vi "Main.vi"() -> ()   [LabVIEW 2012]
uses:
  <userlib>/DAQNavi Polymorphic VI/create/DAQNavi Create Channel(AI-Voltage).vi
  <userlib>/DAQNavi Polymorphic VI/configure/timing/DAQNavi Timing(AI Convert Clock).vi
  <userlib>/DAQNavi Polymorphic VI/read/DAQNavi Read (Analog 1D U16 NChan NSamp).vi
panel:
  out "y aixs max":dbl
  out "y aixs min":dbl
  in  "device module":string="DemoDevice,BID#0/module0" caption="device"
  out "read buffer size":u32
  out "channel count":i32
  out "convert rate":dbl
  out "Acquisition Szie":u64
  out "waveform chart":waveform(u16)[](graph)
  in  "Disable Buffering? (T)":bool=TRUE caption="禁用缓冲？(T)"
  in  "number of samples per channel to read":u32=131072
  out "overrun count":i32
  in  "File Path":path=path "c:/labview/data/data.tdms"
  out "value range":string="+/- 5 V" caption="property value"
  out "physical channels":string="DemoDevice,BID#0/ai0:0" caption="property value"
  in  "samples per channel":u32=131072
  out "actual convert rate":dbl
  in  "convert clock rate":dbl=100000000.0
  in  "start acq":bool
  in  "stop acq":bool
  in  "stop read":bool
  in  "read flag":bool
  in  "acq flag":bool
  in  "start read":bool
  in  "exist":bool
  # "Please modify physical channels and value range in Channel Parameters through DAQNavi Property Assistant VI  in block diagram.\nPlease modify the file path before  save / read data.\n\nThis example is used to  show how to save data when convert clock rate  more than 1M. In order to improve the storage efficiency,the acquisition data is raw data in this example, if you want save data when  convert clock rate  less than 1M, you can use the scale data."
  # "Channel Parameters"
  # "Replay"
  # "Acquisition"
  # "Timing Parameters"
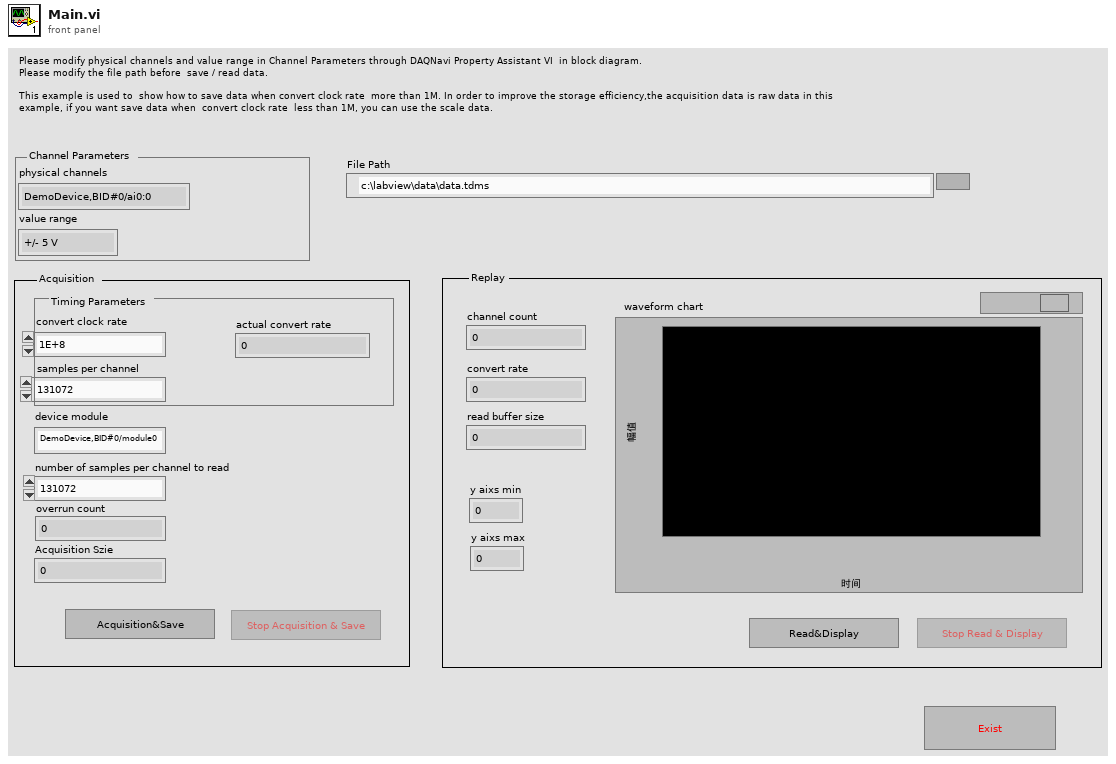
[diagram p1: front panel]
types:
  T1 = enum8{"Enabled", "Disabled", "Disabled and Grayed Out"}
  T2 = cluster{" rate":dbl, "channel count":i32, "min":dbl, "max":dbl, "resolution":i32, "data mask":i32}
  T3 = enum16{"open", "open or create", "create or replace", "create", "open (read-only)"}
  T4 = cluster{"rate":dbl, "section length":u32, "channel count":u32, "y min":dbl, "y max":dbl, "multiplier":dbl}
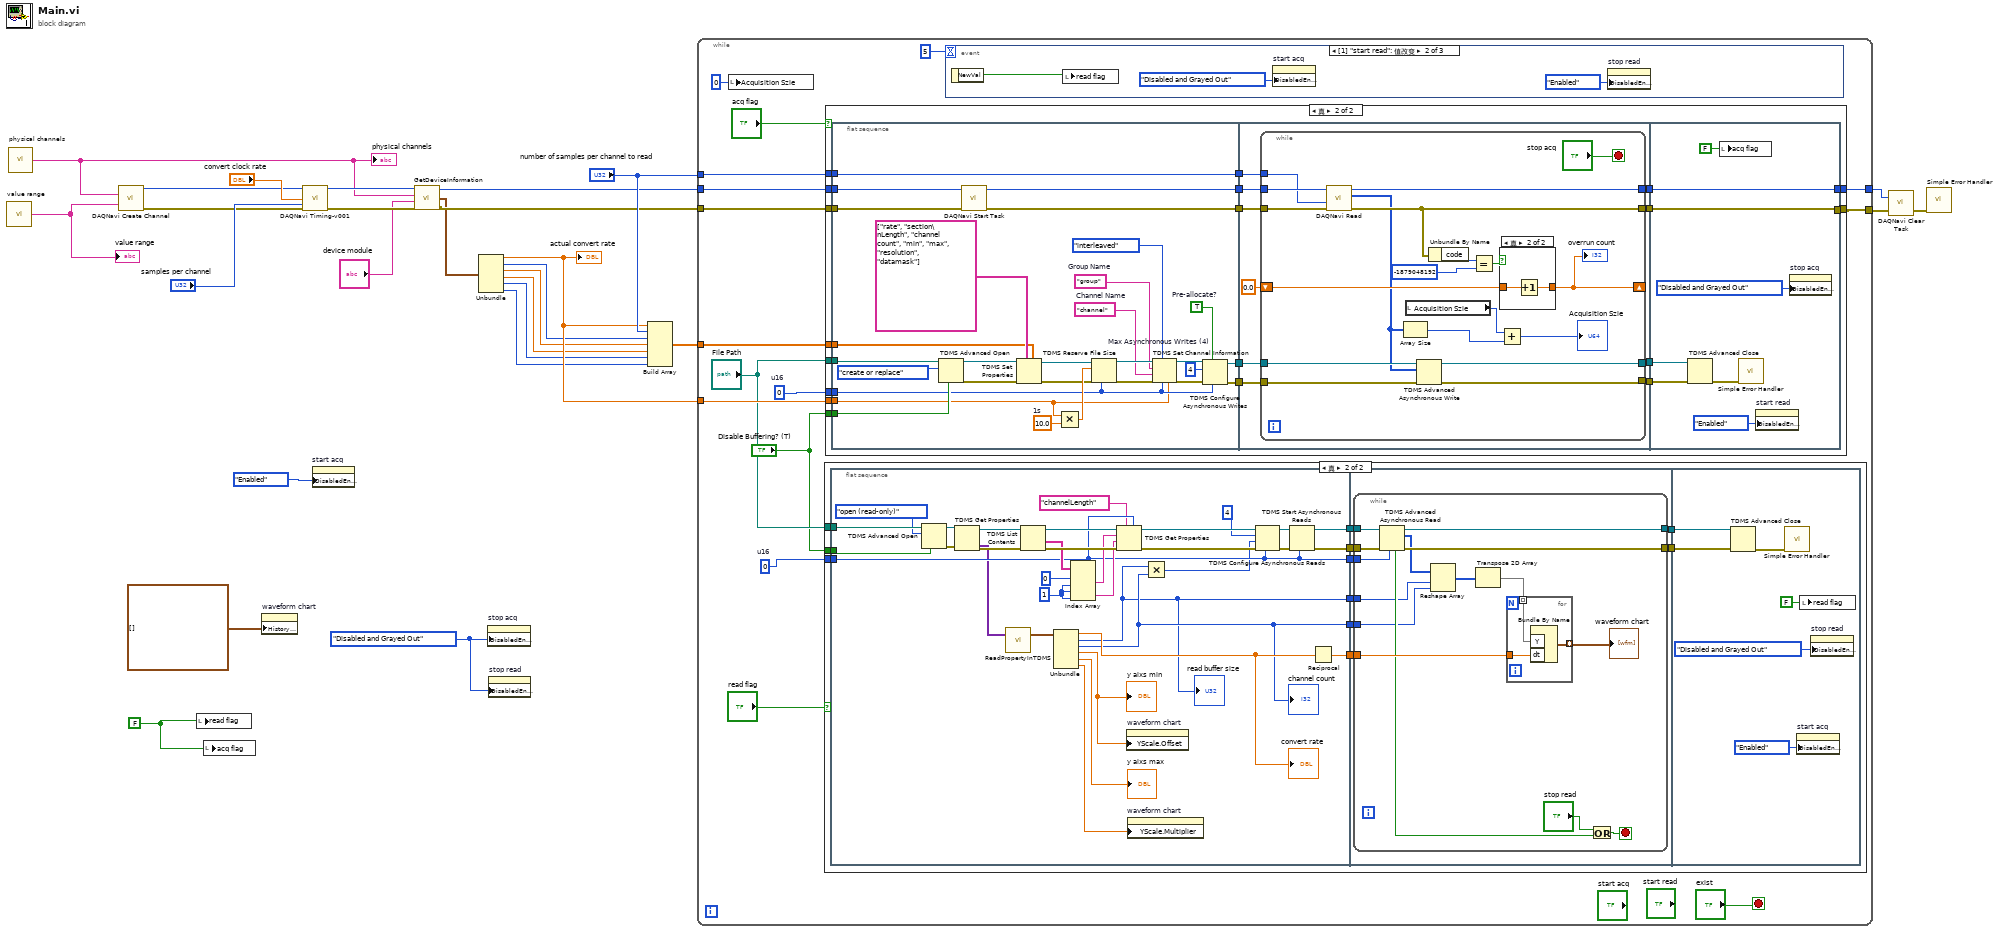
[diagram p0: block diagram]
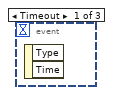
[diagram p5: hidden frame]
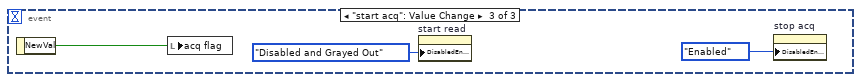
[diagram p6: hidden frame]
diagram:
  w19 = T1."Disabled and Grayed Out" ("禁用")
  w23 = FALSE ("read flag")
  n1 = call "value range"() -> ("property value"=w17:string)  [unwired: 1 out]
  "value range" <- w17
  n2 = call "physical channels"() -> ("property value"=w3:string)  [unwired: 1 out]
  "physical channels" <- w3
  n3 = call-poly <userlib>:"DAQNavi Create Channel.vi"("physical channels"=w3, "value range"=w17) -> ("task out"=w15:i32, "error out"=w16:errorcluster)  [unwired: 3 in, 9 out]
  n4 = local write "read flag"(w23) -> ()
  n5 = local write "acq flag"(w23) -> ()
  n6 = property on="waveform chart" class="WFChart (严格)"("History Data"=waveform(u16)[][] [] ("历史数据")) -> ()  [unwired: 2 in, 2 out]
  n7 = call-poly <userlib>:"DAQNavi Timing-v001.vi"("task in"=w15, "rate"="convert clock rate", "section length"="samples per channel", "error in (no error)"=w16) -> ("task out"=w14:i32, "error out"=w13:errorcluster)  [unwired: 3 in, 7 out]
  n8 = property on="start acq" class="Bool"("DisabledEnum"=T1."Enabled" ("禁用")) -> ()  [unwired: 2 in, 2 out]
  n9 = call "GetDeviceInformation.vi"("error in (no error)"=w13, "device module"="device module", "physical channels"=w3, "task in"=w14) -> ("错误输出"=w10:errorcluster, "输出簇"=w9:T2, "task out"=w11:i32)
  n10 = Unbundle(w9) -> ("rate"=w8:dbl, "channel count"=w7:i32, "min"=w2:dbl, "max"=w6:dbl, "resolution"=w5:i32, "data mask"=w4:i32)
  "actual convert rate" <- w8
  n11 = property on="stop acq" class="Bool"("DisabledEnum"=w19) -> ()  [unwired: 2 in, 2 out]
  n12 = property on="stop read" class="Bool"("DisabledEnum"=w19) -> ()  [unwired: 2 in, 2 out]
  n13 = Build Array(w8, "number of samples per channel to read", w7, w2, w6, w5, w4) -> (w20:dbl[])
  n14 = while {
    tunnel: w11 -> [w39]
    tunnel: w10 -> [w38]
    tunnel: w8 -> [w35]
    tunnel: [w37] -> w24
    tunnel: [w36] -> w25
    tunnel: "number of samples per channel to read" -> [w34]
    tunnel: w20 -> [w30]
    stop <- "exist" stop-if-true
    w28 = u16 0  # u16
    w33 = u16 0  # u16
    n15 = local write "Acquisition Szie"(0 ("Acquisition Szie")) -> ()
    n16 = case shown="真" "read flag" {
      tunnel: "File Path" -> [_ w54]
      tunnel: "Disable Buffering? (T)" -> [_ w53]
      tunnel: w28 -> [_ w52]
      frame False {
      }
      frame True {
        n17 = flat-sequence {
          tunnel: w54 -> [w87]
          tunnel: w53 -> [w85]
          tunnel: w52 -> [w70]
          tunnel: [w74] -> w51
          tunnel: [w71] -> w50
          tunnel: [w70] -> w49
          tunnel: [w64] -> w48
          tunnel: [w59] -> w45
          tunnel: [w55] -> w44
          tunnel: w51 -> [w95]
          tunnel: w50 -> [w94]
          tunnel: w49 -> [w93]
          tunnel: w48 -> [w92]
          tunnel: [w91] -> w47
          tunnel: [w90] -> w46
          tunnel: w45 -> [w89]
          tunnel: w44 -> [w88]
          tunnel: w47 -> [w118]
          tunnel: w46 -> [w117]
          frame #0 {
            w78 = 1 ("禁用的索引 (列)")
            n18 = TDMS Advanced Open(6:w85, 10:T3."open (read-only)" ("操作(0:open)"), 11:w87) -> (0:w67:errorcluster, 3:w68:refnum<k34>)  [unwired: 2 in, 1 out]
            n19 = TDMS Get Properties(8:w67, 11:w68) -> (0:w65:errorcluster, 3:w66:refnum<k34>, 4:w61:variant[])  [unwired: 4 in, 3 out]
            n20 = call "ReadPropertyInTDMS.vi"("数组"=w61) -> ("输出簇"=w62:T4)  [unwired: 2 in]
            n21 = TDMS List Contents(4:w65, 7:w66) -> (0:w84:errorcluster, 1:w80:string[][], 3:w82:refnum<k34>)  [unwired: 1 in, 1 out]
            n22 = Unbundle(w62) -> ("rate"=w60:dbl, "section length"=w55:u32, "channel count"=w59:u32, "y min"=w57:dbl, "y max"=→"y aixs max":dbl, "multiplier"=w58:dbl)
            "convert rate" <- w60
            "channel count" <- w59
            "read buffer size" <- w55
            "y aixs min" <- w57
            n23 = Index Array(array=w80, index (row) #1=0 ("索引 (行)"), index (col) #1=w78, index (row) #2=w78, index (col) #2=w78) -> (element #1=w77:string, element #2=w76:string)
            n24 = TDMS Get Properties(5:w70, 7:"channelLength" ("属性名称"), 8:w84, 9:w76, 10:w77, 11:w82) -> (0:w83:errorcluster, 3:w81:refnum<k34>)  [unwired: 4 out]
            n25 = property on="waveform chart" class="WFChart (严格)"("YScale.Offset"=w57) -> ()  [unwired: 2 in, 2 out]
            n26 = property on="waveform chart" class="WFChart (严格)"("YScale.Multiplier"=w58) -> ()  [unwired: 2 in, 2 out]
            n27 = Multiply(x=w55, y=w59) -> (x*y=w63:u32)
            n28 = TDMS Configure Asynchronous Reads(6:w70, 8:w83, 9:w63, 10:u32 4 ("缓冲区数量(4)"), 11:w81) -> (0:w72:errorcluster, 3:w73:refnum<k34>)  [unwired: 1 in]
            n29 = TDMS Start Asynchronous Reads(6:w70, 8:w72, 11:w73) -> (0:w71:errorcluster, 3:w74:refnum<k34>)  [unwired: 1 in]
            n30 = Reciprocal(x=w60) -> (1/x=w64:dbl)
          }
          frame #1 {
            n31 = while {
              tunnel: w95 -> [w110]
              tunnel: w94 -> [w109]
              tunnel: w93 -> [w108]
              tunnel: w92 -> [w105]
              tunnel: [w104] -> w91
              tunnel: [w103] -> w90
              tunnel: w89 -> [w98]
              tunnel: w88 -> [w97]
              stop <- w107 stop-if-true
              n32 = TDMS Advanced Asynchronous Read(6:w108, 8:w109, 11:w110) -> (0:w103:errorcluster, 2:w99:u16[], 3:w104:refnum<k34>, 4:w102:bool)
              n33 = Reshape Array(w99, w97, w98) -> (w100:u16[][])
              n34 = Transpose 2D Array(2D array=w100) -> (transposed array=w101:u16[][])
              n35 = for {
                tunnel: [w113] -> w106 mode=indexing
                tunnel: w105 -> [w111]
                tunnel: w101 -> [w112] mode=indexing
                n36 = Bundle By Name("Y"=w112, "dt"=w111) -> (w113:waveform(u16))  [unwired: 1 in]
              }
              "waveform chart" <- w106
              n37 = Or(x="stop read", y=w102) -> (x .or. y?=w107:bool)
            }
          }
          frame #2 {
            n38 = TDMS Advanced Close(8:w117, 11:w118) -> (0:w114:errorcluster)  [unwired: 2 in, 1 out]
            n39 = call <vilib>:"Simple Error Handler.vi"("error in (no error)"=w114) -> ()  [unwired: 4 in, 5 out]
            n40 = property on="start acq" class="Bool"("DisabledEnum"=T1."Enabled" ("禁用")) -> ()  [unwired: 2 in, 2 out]
            n41 = local write "read flag"(FALSE ("read flag")) -> ()
            n42 = property on="stop read" class="Bool"("DisabledEnum"=T1."Disabled and Grayed Out" ("禁用")) -> ()  [unwired: 2 in, 2 out]
          }
        }
      }
    }
    n43 = case shown="真" "acq flag" {
      tunnel: w39 -> [w121 w140]
      tunnel: w38 -> [w120 w139]
      tunnel: w35 -> [_ w138]
      tunnel: "File Path" -> [_ w137]
      tunnel: [w120 w129] -> w37
      tunnel: [w121 w127] -> w36
      tunnel: "Disable Buffering? (T)" -> [_ w126]
      tunnel: w33 -> [_ w125]
      tunnel: w34 -> [_ w124]
      tunnel: w30 -> [_ w122]
      frame False {
      }
      frame True {
        n44 = flat-sequence {
          tunnel: w140 -> [w169]
          tunnel: w139 -> [w168]
          tunnel: w138 -> [w148]
          tunnel: w137 -> [w156]
          tunnel: [w155] -> w136
          tunnel: [w154] -> w135
          tunnel: [w153] -> w132
          tunnel: [w152] -> w131
          tunnel: w126 -> [w151]
          tunnel: w125 -> [w150]
          tunnel: w124 -> [w149]
          tunnel: [w149] -> w123
          tunnel: w122 -> [w141]
          tunnel: w136 -> [w179]
          tunnel: w135 -> [w178]
          tunnel: [w177] -> w134
          tunnel: [w176] -> w133
          tunnel: w132 -> [w175]
          tunnel: w131 -> [w174]
          tunnel: [w173] -> w130
          tunnel: [w172] -> w128
          tunnel: w123 -> [w171]
          tunnel: w134 -> [w208]
          tunnel: w133 -> [w204]
          tunnel: w130 -> [w202]
          tunnel: [w202] -> w129
          tunnel: w128 -> [w207]
          tunnel: [w207] -> w127
          frame #0 {
            w147 = 10.0  # 1s
            w159 = "channel"  # Channel Name
            w160 = "group"  # Group Name
            w161 = u32 4  # Max Asynchronous Writes (4)
            w162 = TRUE  # Pre-allocate?
            n45 = TDMS Advanced Open(6:w151, 10:T3."create or replace" ("操作(0:open)"), 11:w156) -> (0:w144:errorcluster, 3:w146:refnum<k34>)  [unwired: 2 in, 1 out]
            n46 = call <userlib>:"DAQNavi Start Task.vi"("error in (no error)"=w168, "task in"=w169) -> ("error out"=w152:errorcluster, "task out"=w153:i32)  [unwired: 8 in]
            n47 = TDMS Set Properties(5:w141, 7:string[] ["rate", "section\nLength", "channel count", "min", "max", "resolution", "datamask"] ("属性名称"), 8:w144, 11:w146) -> (0:w143:errorcluster, 3:w145:refnum<k34>)  [unwired: 2 in, 2 out]
            n48 = Multiply(x=w148, y=w147) -> (x*y=w158:dbl)
            n49 = TDMS Reserve File Size(6:w150, 8:w143, 10:w158, 11:w145) -> (0:w166:errorcluster, 3:w165:refnum<k34>)  [unwired: 1 in]
            n50 = TDMS Set Channel Information(4:w148, 6:w150, 7:enum16{"non-interleaved", "interleaved"}."interleaved" ("数据布局（0:非交叉）"), 8:w166, 9:w159, 10:w160, 11:w165) -> (0:w163:errorcluster, 3:w164:refnum<k34>)
            n51 = TDMS Configure Asynchronous Writes(6:w150, 7:w162, 8:w163, 10:w161, 11:w164) -> (0:w154:errorcluster, 3:w155:refnum<k34>)  [unwired: 2 in]
          }
          frame #1 {
            n52 = while {
              tunnel: w179 -> [w198]
              tunnel: w178 -> [w197]
              tunnel: [w196] -> w177
              tunnel: [w195] -> w176
              shift-right: [w190] -> _
              shift-left: 0.0 -> [w191]
              tunnel: w175 -> [w189]
              tunnel: w174 -> [w188]
              tunnel: [w187] -> w173
              tunnel: [w186] -> w172
              tunnel: w171 -> [w185]
              stop <- "stop acq" stop-if-true
              n53 = call-poly <userlib>:"DAQNavi Read.vi"("error in (no error)"=w188, "number of samples per channel to read"=w185, "task in"=w189) -> ("error out"=w187:errorcluster, "data"=w184:u16[], "task out"=w186:i32)  [unwired: 1 in, 5 out]
              n54 = Array Size(array=w184) -> (size(s)=w182:i32)
              n55 = local read "Acquisition Szie"() -> (w183:u64)
              n56 = TDMS Advanced Asynchronous Write(8:w197, 10:w184, 11:w198) -> (0:w195:errorcluster, 3:w196:refnum<k34>)
              n57 = Unbundle By Name(w187) -> ("code"=w193:i32)
              n58 = Equal?(x=w193, y=-1879048192) -> (x = y?=w194:bool)
              n59 = case shown="真" w194 {
                tunnel: w191 -> [w199 w201]
                tunnel: [w199 w200] -> w190
                frame False {
                }
                frame True {
                  n60 = Increment(x=w201) -> (x+1=w200:dbl)
                }
              }
              "overrun count" <- w190
              n61 = Add(x=w183, y=w182) -> (x+y=→"Acquisition Szie":u64)
            }
          }
          frame #2 {
            n62 = TDMS Advanced Close(8:w204, 11:w208) -> (0:w203:errorcluster)  [unwired: 2 in, 1 out]
            n63 = local write "acq flag"(FALSE ("acq flag")) -> ()
            n64 = call <vilib>:"Simple Error Handler.vi"("error in (no error)"=w203) -> ()  [unwired: 4 in, 5 out]
            n65 = property on="start read" class="Bool"("DisabledEnum"=T1."Enabled" ("禁用")) -> ()  [unwired: 2 in, 2 out]
            n66 = property on="stop acq" class="Bool"("DisabledEnum"=T1."Disabled and Grayed Out" ("禁用")) -> ()  [unwired: 2 in, 2 out]
          }
        }
      }
    }
    n67 = event shown="[1] \"start read\": 值改变" {
      selector: _ -> [_ _ _]
      dyn-events: _ -> [_ _ _]
      timeout: 5 -> [_ _ _]
      event Timeout {
        n68 = event-data() -> ()  [unwired: 1 in, 2 out]
      }
      event "start read": Value Change {
        n69 = event-data() -> ("NewVal"=w212:bool)  [unwired: 1 in]
        n70 = local write "read flag"(w212) -> ()
        n71 = property on="start acq" class="Bool"("DisabledEnum"=T1."Disabled and Grayed Out" ("禁用")) -> ()  [unwired: 2 in, 2 out]
        n72 = property on="stop read" class="Bool"("DisabledEnum"=T1."Enabled" ("禁用")) -> ()  [unwired: 2 in, 2 out]
      }
      event "start acq": Value Change {
        n73 = event-data() -> ("NewVal"=w215:bool)  [unwired: 1 in]
        n74 = local write "acq flag"(w215) -> ()
        n75 = property on="start read" class="Bool"("DisabledEnum"=T1."Disabled and Grayed Out" ("禁用")) -> ()  [unwired: 2 in, 2 out]
        n76 = property on="stop acq" class="Bool"("DisabledEnum"=T1."Enabled" ("禁用")) -> ()  [unwired: 2 in, 2 out]
      }
    }
  }
  n77 = call <userlib>:"DAQNavi Clear Task.vi"("error in (no error)"=w24, "task in"=w25) -> ("error out"=w18:errorcluster)  [unwired: 1 in]
  n78 = call <vilib>:"Simple Error Handler.vi"("error in (no error)"=w18) -> ()  [unwired: 4 in, 5 out]
